vi "fcs_find_data_start.vi"(8 "error in":errorcluster, 11 "File Path":path=path "C:/Users/ignacio/Desktop/Patrick's File Reader Function/snapshot5.fcs") -> (0 "error out":errorcluster, 1 "Number of timepoints":i32, 2 "ENDDATA":i32, 3 "BEGINDATA":i32)   [LabVIEW 2013]
uses:
  <vilib>/regexp/Match Regular Expression.xnode
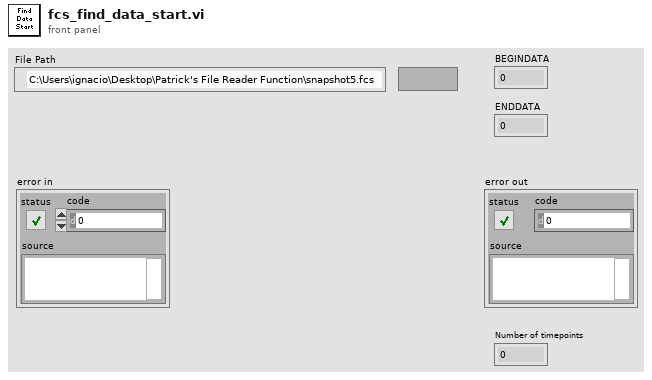
[diagram p1: front panel]
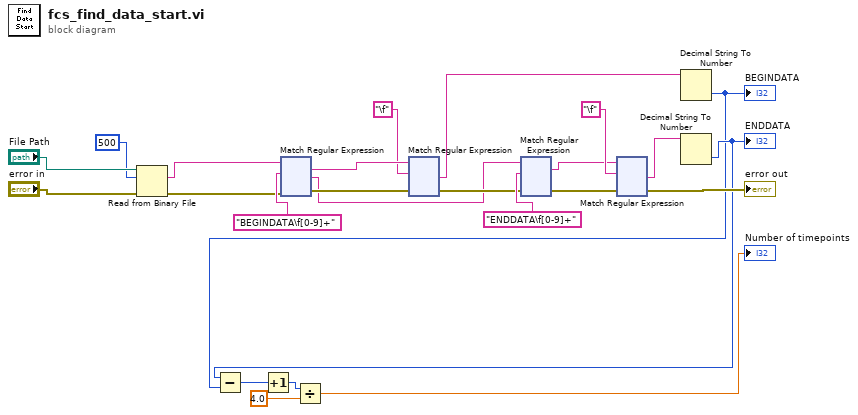
[diagram p0: block diagram]
diagram:
  n1 = Read from Binary File(8:"error in", 10:500 ("Bytes of header to read"), 11:"File Path") -> (0:w20:errorcluster, 2:w18:string)  [unwired: 3 in, 2 out]
  n2 = xnode "Match Regular Expression"("input string"=w18, "regular expression"="BEGINDATA\f[0-9]+", "error in"=w20) -> ("whole match"=w17:string, "after match"=w9:string, "error out"=w15:errorcluster)  [unwired: 3 in, 2 out]
  n3 = xnode "Match Regular Expression"("input string"=w17, "regular expression"="\f", "error in"=w15) -> ("after match"=w7:string, "error out"=w14:errorcluster)  [unwired: 3 in, 3 out]
  n4 = xnode "Match Regular Expression"("input string"=w9, "regular expression"="ENDDATA\f[0-9]+", "error in"=w14) -> ("whole match"=w10:string, "error out"=w12:errorcluster)  [unwired: 3 in, 3 out]
  n5 = xnode "Match Regular Expression"("input string"=w10, "regular expression"="\f", "error in"=w12) -> ("after match"=w8:string, "error out"=→"error out":errorcluster)  [unwired: 3 in, 3 out]
  n6 = Decimal String To Number(string=w7) -> (number=w2:i32)  [unwired: 2 in, 1 out]
  "BEGINDATA" <- w2
  n7 = Decimal String To Number(string=w8) -> (number=w3:i32)  [unwired: 2 in, 1 out]
  "ENDDATA" <- w3
  n8 = Subtract(x=w3, y=w2) -> (x-y=w6:i32)
  n9 = Increment(x=w6) -> (x+1=w5:i32)
  n10 = Divide(x=w5, y=4.0) -> (x/y=→"Number of timepoints":dbl)
